vi "setRampAttributes.vi"(8 "error in (no error)":errorcluster, 9 "Array":string[][](array[string]), 10 "Edit Tree Items:Add Item in":string, 11 "TreeControl in":refnum<vi>) -> (0 "error out":errorcluster, 3 "TreeControl out":refnum<vi>)   [LabVIEW 2021]
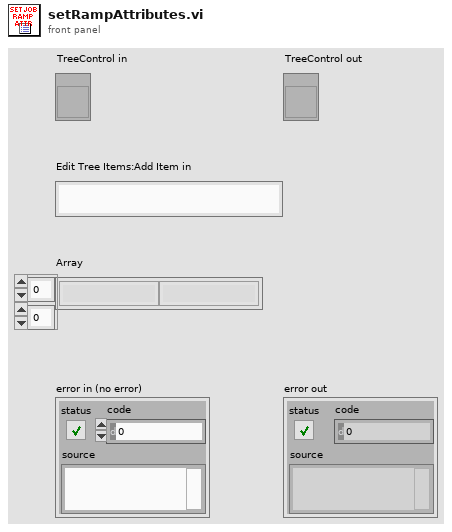
[diagram p1: front panel]
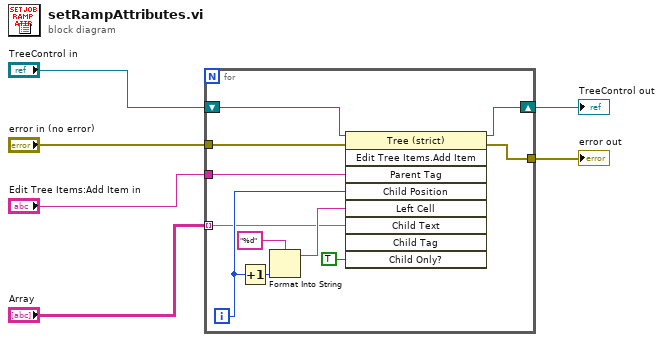
[diagram p0: block diagram]
diagram:
  n1 = for {
    tunnel: "Edit Tree Items:Add Item in" -> [w17]
    tunnel: "error in (no error)" -> [w16]
    tunnel: "Array" -> [w7] mode=indexing
    tunnel: [w15] -> w3
    shift-right: [w13] -> w5
    shift-left: "TreeControl in" -> [w14]
    i -> [w9]
    n2 = Increment(x=w9) -> (x+1=w11:i32)
    n3 = Format Into String(format string="%d", w11) -> (resulting string=w8:string)  [unwired: 2 in, 1 out]
    n4 = invoke on="Invoke Node" class="Tree (strict)" method="Edit Tree Items.Add Item"(reference=w14, error in=w16, "Parent Tag"=w17, "Child Position"=w9, "Left Cell"=w8, "Child Text"=w7, "Child Only?"=TRUE) -> (reference out=w13:refnum<vi>, error out=w15:errorcluster)  [unwired: 2 in, 7 out]
  }
  "TreeControl out" <- w5
  "error out" <- w3
